vi "6 voies.vi"(11 "ECG 2 voies":dbl[][](array[numeric])) -> (3 "ECG à 6 voies":dbl[][](array[numeric]))   [LabVIEW 2017]
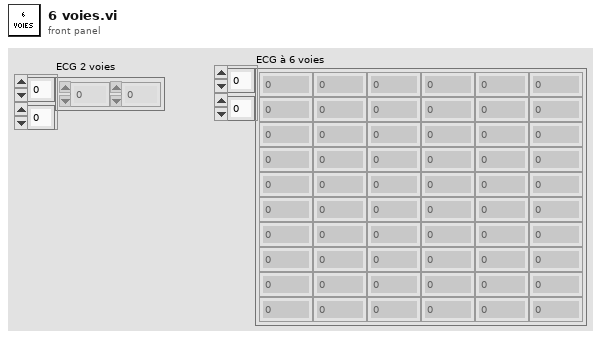
[diagram p1: front panel]
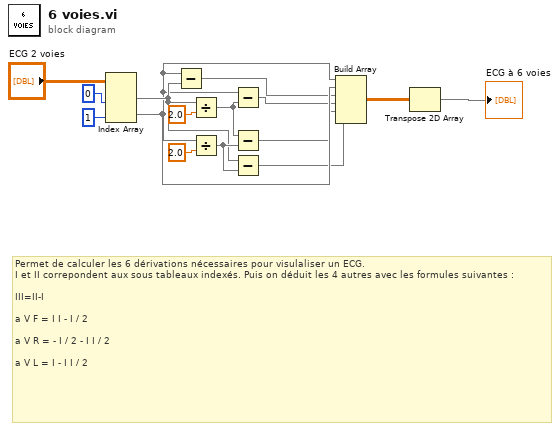
[diagram p0: block diagram]
diagram:
  # "Permet de calculer les 6 dérivations nécessaires pour visulaliser un ECG.\nI et II correpondent aux sous tableaux indexés. Puis on déduit les 4 autres avec les formules suivantes :\n\nIII=II-I\n\na V F = I I - I / 2  \n\na V R = - I / 2 - I I / 2 \n\na V L = I - I I / 2"
  n1 = Index Array(array="ECG 2 voies", index (col) #1=0 ("indice (ligne)"), index (col) #2=1 ("indice désactivé (col)")) -> (element #1=w10:dbl[], element #2=w9:dbl[])  [unwired: 2 in]
  n2 = Subtract(x=w9, y=w10) -> (x-y=w8:dbl[])
  n3 = Divide(x=w10, y=2.0) -> (x/y=w12:dbl[])
  n4 = Divide(x=w9, y=2.0) -> (x/y=w11:dbl[])
  n5 = Subtract(x=w9, y=w12) -> (x-y=w7:dbl[])
  n6 = Subtract(x=w12, y=w11) -> (x-y=w6:dbl[])
  n7 = Subtract(x=w10, y=w11) -> (x-y=w5:dbl[])
  n8 = Build Array(w9, w9, w8, w7, w6, w5) -> (w4:dbl[][])
  n9 = Transpose 2D Array(2D array=w4) -> (transposed array=→"ECG à 6 voies":dbl[][])
